vi "SetupKeithley.vi"(4 "Enable Resistance Auto Range (T:Enable)":bool=TRUE, 5 "Serial Configuration":T1={"Baud Rate"=9600, "Parity"=0, "Data Bits"=8, "Stop Bits"=10, "Flow Control"=0} {"Flow Control" items=["None", "XON/XOFF", "RTS/CTS", "XON/XOFF & RTS/CTS", "DTR/DSR", "XON/XOFF & DTR/DSR"]; "Stop Bits" items=["1.0"=10, "1.5"=15, "2.0"=20]; "Data Bits" items=["7"=7, "8"=8]; "Parity" items=["None", "Odd", "Even", "Mark", "Space"]; "Baud Rate" items=["300"=300, "600"=600, "1200"=1200, "2400"=2400, "4800"=4800, "9600"=9600, "19200"=19200]}, 6 "Current Manual Range (1.0)":dbl=1.0, 7 "Enable Voltage Auto Range (T:Enable)":bool=TRUE, 8 "Enable Current Auto Range (T:Enable)":bool=TRUE, 9 "Resistance Manual Range (1.0)":dbl=1.0, 10 "Voltage Manual Range (1.0)":dbl=1.0, 11 "VISA Refnum in":refnum<visa-resource-name>) -> (0 "error out":errorcluster, 3 "VISA Refnum out":refnum<visa-resource-name>)   [LabVIEW 2013]
uses:
  <instrlib>/Keithley 24XX/Keithley 24XX.lvlib
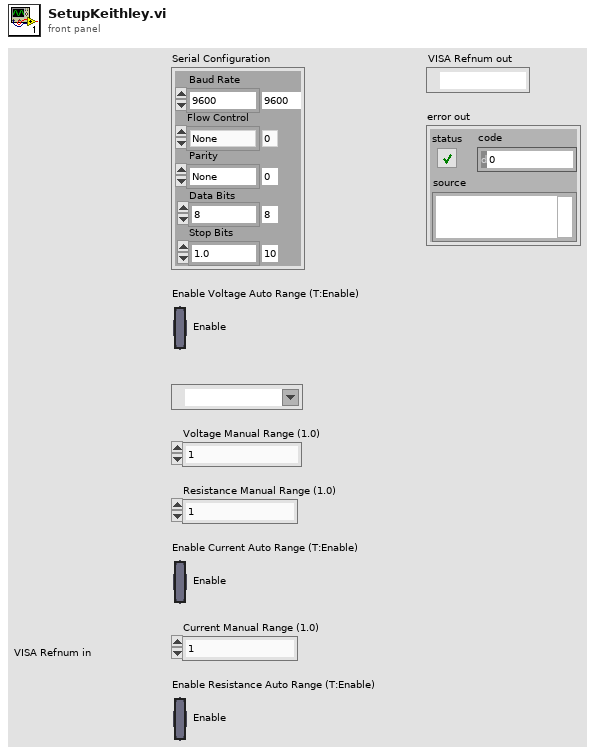
[diagram p1: front panel]
types:
  T1 = cluster{"Baud Rate":u32, "Parity":u16, "Data Bits":u16, "Stop Bits":u16, "Flow Control":u16}
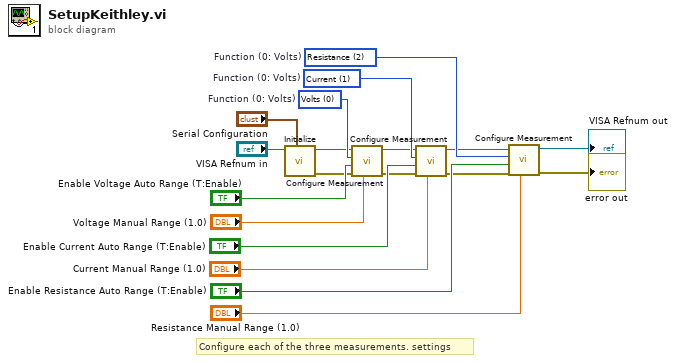
[diagram p0: block diagram]
diagram:
  w11 = u16 2 items=["Volts", "Current", "Resistance"]  # Function (0: Volts)
  w10 = u16 1 items=["Volts", "Current", "Resistance"]  # Function (0: Volts)
  w9 = u16 0 items=["Volts", "Current", "Resistance"]  # Function (0: Volts)
  # "Configure each of the three measurements. settings"
  n1 = call <instrlib>:"Initialize.vi"("Serial Configuration"="Serial Configuration", "VISA resource name"="VISA Refnum in") -> ("error out"=w4:errorcluster, "VISA resource name out"=w3:refnum<visa-resource-name>)  [unwired: 8 in]
  n2 = call <instrlib>:"Configure Measurement.vi"("Manual Range (1.0)"="Voltage Manual Range (1.0)", "error in (no error)"=w4, "Enable Auto Range (T:Enable)"="Enable Voltage Auto Range (T:Enable)", "Function (0: Volts)"=w9, "VISA resource name"=w3) -> ("error out"=w6:errorcluster, "VISA resource name out"=w5:refnum<visa-resource-name>)  [unwired: 5 in]
  n3 = call <instrlib>:"Configure Measurement.vi"("Manual Range (1.0)"="Current Manual Range (1.0)", "error in (no error)"=w6, "Enable Auto Range (T:Enable)"="Enable Current Auto Range (T:Enable)", "Function (0: Volts)"=w10, "VISA resource name"=w5) -> ("error out"=w7:errorcluster, "VISA resource name out"=w8:refnum<visa-resource-name>)  [unwired: 5 in]
  n4 = call <instrlib>:"Configure Measurement.vi"("Manual Range (1.0)"="Resistance Manual Range (1.0)", "error in (no error)"=w7, "Enable Auto Range (T:Enable)"="Enable Resistance Auto Range (T:Enable)", "Function (0: Volts)"=w11, "VISA resource name"=w8) -> ("error out"=→"error out":errorcluster, "VISA resource name out"=→"VISA Refnum out":refnum<visa-resource-name>)  [unwired: 5 in]
